vi "Do.vi"(8 "error in (no error)":errorcluster, 10 "Actor in":refnum<class "Actor.lvclass">, 11 "Conceret Test Node Next Button Visibility Msg in":refnum<class "Conceret Test Node Next Button Visibility Msg.lvclass">) -> (0 "error out":errorcluster, 2 "Actor out":refnum<class "Actor.lvclass">)   [LabVIEW 2013, in "Test Node View.lvlib" / "Conceret Test Node Next Button Visibility Msg.lvclass"]
doc: "(<B>Filename</B>: Actor Framework.lvlib:Message.lvclass:Do.vi)\n\nDefines what a message does when it is received by an actor. Generally, a message instructs an actor to invoke one of its methods.\n\nBy default, this method does nothing. A child class must override it to define behavior. Create a child class by using the Actor Framework Message Maker dialog box."
uses:
  Conceret Test Node Next Button Visibility Msg.lvclass
  <vilib>/ActorFramework/Actor/Actor.lvclass
  Test Node View/Test Node View.lvclass
  Models/Test Node Model Messages/Abstract Test Node Next Button Visibility Msg/Abstract Test Node Next Button Visibility Msg.lvclass
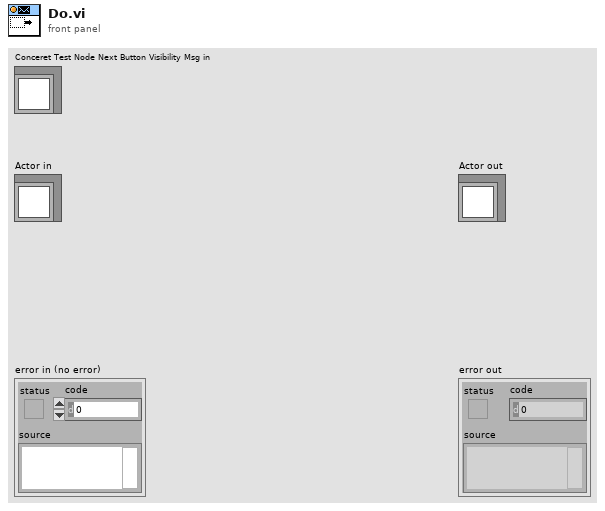
[diagram p1: front panel]
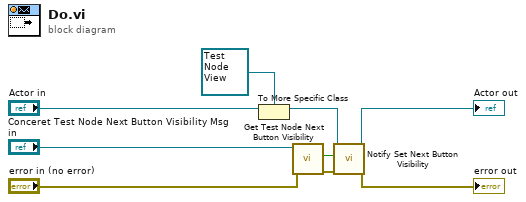
[diagram p0: block diagram]
diagram:
  n1 = To More Specific Class(target class=refnum<class "Test Node View.lvclass"> refnum ("Test Node View.lvlib:Test Node View.lvclass"), reference="Actor in") -> (specific class reference=w6:refnum<class "Test Node View.lvclass">)  [unwired: 1 in, 1 out]
  n2 = call "Get Test Node Next Button Visibility.vi"("error in (no error)"="error in (no error)", "Abstract Test Node Next Button Visibility Msg in"="Conceret Test Node Next Button Visibility Msg in") -> ("error out"=w5:errorcluster, "Test Node Next Button Visibility"=w1:bool)  [unwired: 7 in, 1 out]
  n3 = call "Notify Set Next Button Visibility.vi"("error in (no error)"=w5, "Test Node Next Button Visibility"=w1, "Test Node View in"=w6) -> ("error out"=→"error out":errorcluster, "Test Node View out"=→"Actor out":refnum<class "Test Node View.lvclass">)  [unwired: 7 in]
